vi "UART Read.vi"(8 "Error In":errorcluster, 9 "Num Bytes":u8, 10 "UART Channel (0)":u8, 11 "LINX Resource":T1) -> (0 "Error Out":errorcluster, 2 "Data":u8[](array[numeric]), 3 "LINX Resource":T1)   [LabVIEW 2013, in "LVH-LINX.lvlib"]
doc: "Read the specified number of bytes from the specified UART channel's receive buffer."
uses:
  <vilib>/LabVIEW Hacker/LINX/LVH-LINX.lvlib
  <vilib>/LabVIEW Hacker/LINX/Private/Type Defs/LINX Ref.ctl
  <vilib>/LabVIEW Hacker/LINX/Private/Type Defs/Platform.ctl
  <vilib>/LabVIEW Hacker/LINX/Private/Type Defs/Interface.ctl
  <vilib>/LabVIEW Hacker/LINX/Private/Device/Type Defs/LINX Device Config.ctl
  <vilib>/LabVIEW Hacker/LINX/Private/Device/Type Defs/TCP Config.ctl
  <vilib>/LabVIEW Hacker/LINX/Private/Type Defs/Device Family.ctl
  <vilib>/LabVIEW Hacker/LINX/Private/Type Defs/Peripheral.ctl
  <vilib>/LabVIEW Hacker/LINX/Private/Type Defs/Channel FGV States.ctl
  <vilib>/LabVIEW Hacker/LINX/Private/Device/Device.lvlib
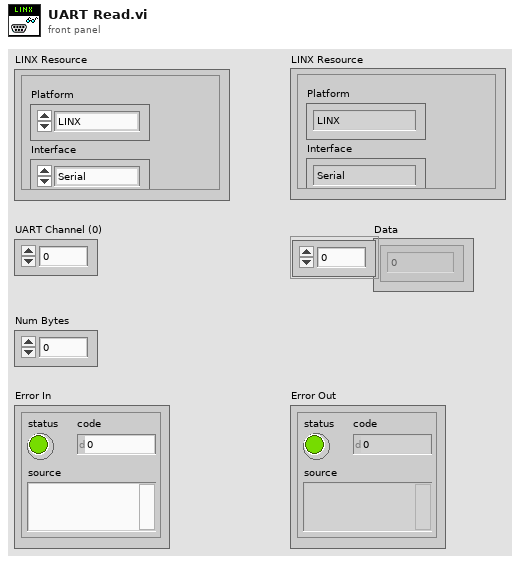
[diagram p1: front panel]
types:
  T1 = typedef "LVH-LINX.lvlib/LINX Ref.ctl" = cluster{"Platform":T2, "Interface":T3, "LINX Device Config":T4}
  T2 = typedef "LVH-LINX.lvlib/Platform.ctl" = enum16{"LINX", "myRIO"}
  T3 = typedef "LVH-LINX.lvlib/Interface.ctl" = enum16{"Serial", "TCP"}
  T4 = typedef "LVH-LINX.lvlib/Device.lvlib/LINX Device Config.ctl" = cluster{"Interface":T3, "COM Port":refnum<visa-resource-name>, "TCP Configuration":T5, "Device Family":T6, "Device ID":u8, "Device Name":string, "TCP Ref":refnum<k5>}
  T5 = typedef "LVH-LINX.lvlib/Device.lvlib/TCP Config.ctl" = cluster{"IP Address":string, "Port":u16}
  T6 = typedef "LVH-LINX.lvlib/Device Family.ctl" = enum8{"National Instruments", "Digilent", "Arduino"}
  T7 = typedef "LVH-LINX.lvlib/Peripheral.ctl" = enum8{"DI", "DO", "AI", "AO", "PWM", "QE", "UART", "I2C", "SPI", "CAN"}
  T8 = typedef "LVH-LINX.lvlib/Channel FGV States.ctl" = enum16{"Initialize", "Get", "Set"}
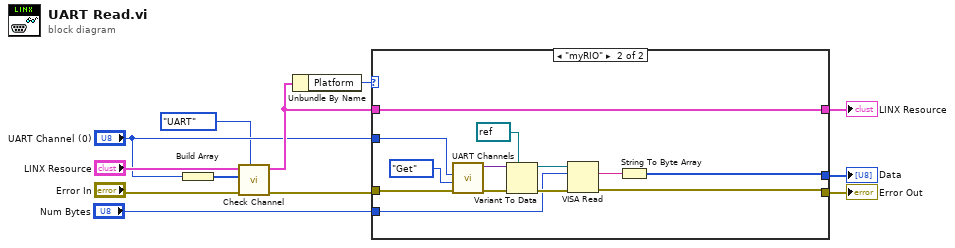
[diagram p0: block diagram]
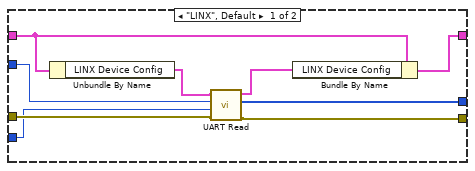
[diagram p2: hidden frame]
diagram:
  n1 = Build Array("UART Channel (0)") -> (w5:u8[])
  n2 = call <vilib>:"Check Channel.vi"("Peripheral"=Peripheral."UART", "Error In"="Error In", "Channels"=w5, "LINX Resource"="LINX Resource") -> ("Error Out"=w6:errorcluster, "LINX Resource"=w7:T1)  [unwired: 5 in, 1 out]
  n3 = Unbundle By Name(w7) -> ("Platform"=w12:T2)
  n4 = case shown="\"myRIO\"" w12 {
    tunnel: w6 -> [w18 w33]
    tunnel: w7 -> [w21 w34]
    tunnel: [w19 w25] -> w11
    tunnel: [w20 w34] -> w10
    tunnel: "UART Channel (0)" -> [w14 w29]
    tunnel: [w15 w22] -> w1
    tunnel: "Num Bytes" -> [w13 w24]
    frame "LINX", Default {
      n5 = Unbundle By Name(w21) -> ("LINX Device Config"=w17:T4)
      n6 = call <vilib>:"UART Read.vi"("Error In"=w18, "Num Bytes"=w13, "UART Channel"=w14, "LINX Device Config"=w17) -> ("Error Out"=w19:errorcluster, "Data"=w15:u8[], "LINX Device Config"=w16:T4)  [unwired: 5 in]
      n7 = Bundle By Name(cluster=w21, "LINX Device Config"=w16) -> (w20:T1)
    }
    frame "myRIO" {
      n8 = call <vilib>:"UART Channels.vi"("Error In"=w33, "Channel State"=Channel_FGV_States."Get", "Channel Number"=w29) -> ("Error Out"=w32:errorcluster, "UART Channel"=w31:variant)  [unwired: 7 in]
      n9 = Variant To Data(error in=w32, type=refnum<visa-resource-name> refnum ("reference"), Variant=w31) -> (data=w27:refnum<visa-resource-name>, error out=w26:errorcluster)
      n10 = VISA Read(VISA resource name=w27, byte count=w24, error in (no error)=w26) -> (read buffer=w23:string, error out=w25:errorcluster)  [unwired: 2 out]
      n11 = String To Byte Array(string=w23) -> (unsigned byte array=w22:u8[])
    }
  }
  "Error Out" <- w11
  "LINX Resource" <- w10
  "Data" <- w1
